vi "Redraw graphs.vi"(6 "Data":sgl[][](array[numeric]), 8 "error in (no error)":errorcluster, 9 "Selected exp":bool=TRUE, 10 "ChangeAll":bool, 11 "Control-Client in":refnum<class "Control-Client.lvclass">) -> (0 "error out":errorcluster, 3 "Control-Client out":refnum<class "Control-Client.lvclass">)   [LabVIEW 2018, in "Control-Client.lvclass"]
uses:
  Control-Client.lvclass
  Control-Client.lvclass/Control-Client.ctl
  Experiments/Experiment.lvclass
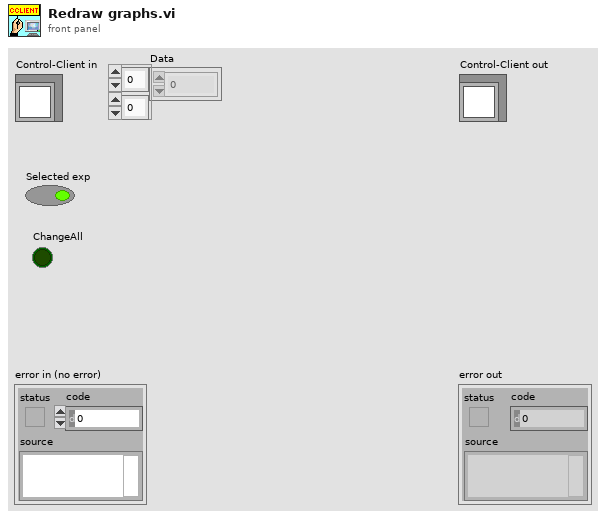
[diagram p1: front panel]
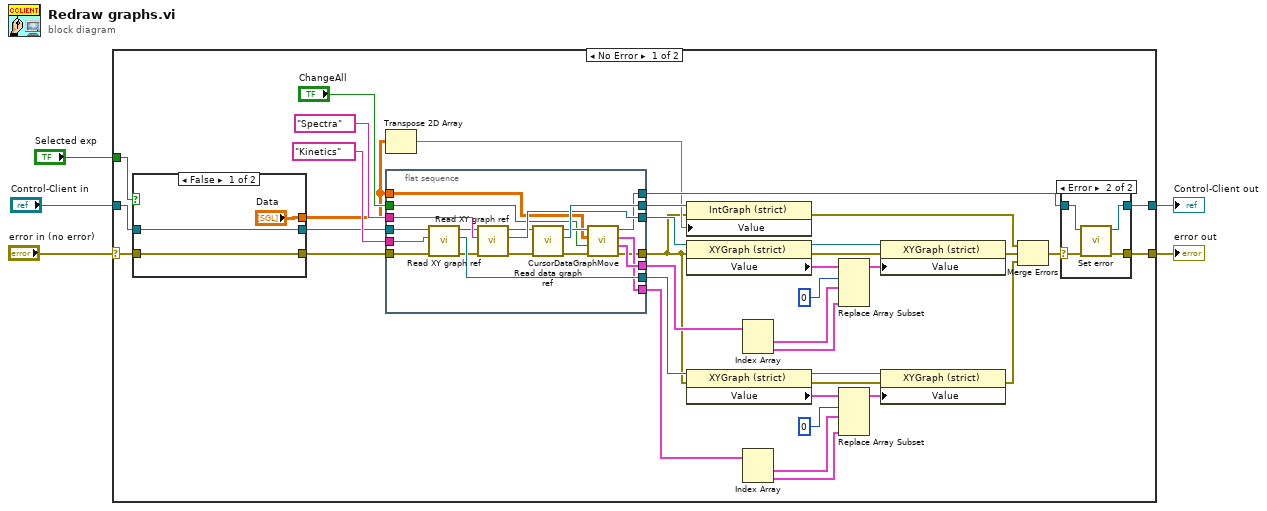
[diagram p0: block diagram]
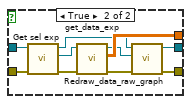
[diagram p2: hidden frame]
diagram:
  n1 = case shown="No Error" "error in (no error)" {
    selector: "error in (no error)" -> [w16 w82]
    tunnel: [w13 w81] -> w3
    tunnel: "Control-Client in" -> [w17 w81]
    tunnel: [w11 w82] -> w2
    tunnel: "Selected exp" -> [w10 _]
    frame No Error {
      n2 = case shown="False" w10 {
        tunnel: w17 -> [w44 w55]
        tunnel: w16 -> [w45 w54]
        tunnel: [w45 w50] -> w6
        tunnel: ["Data" w52] -> w8
        tunnel: [w44 w49] -> w15
        frame False {
        }
        frame True {
          n3 = call "Get sel exp.vi"("error in (no error)"=w54, "Control-Client in"=w55) -> ("error out"=w53:errorcluster, "Sel experiment"=w51:refnum<class "Experiment.lvclass">, "Control-Client out"=w46:refnum<class "Control-Client.lvclass">)  [unwired: 7 in]
          n4 = call "get_data_exp.vi"("error in (no error)"=w53, "Experiment.lvclass in"=w51) -> ("error out"=w47:errorcluster, "Data"=w52:sgl[][], "Experiment.lvclass out"=w48:refnum<class "Experiment.lvclass">)  [unwired: 7 in]
          n5 = call "Redraw_data_raw_graph.vi"("error in (no error)"=w47, "Sel experiment"=w48, "Control-Client in"=w46) -> ("error out"=w50:errorcluster, "Control-Client out"=w49:refnum<class "Control-Client.lvclass">)  [unwired: 7 in]
        }
      }
      n6 = Transpose 2D Array(2D array=w8) -> (transposed array=w9:sgl[][])
      n7 = flat-sequence {
        tunnel: "Kinetics" ("Combo Box") -> [w80]
        tunnel: "Spectra" ("Combo Box") -> [w79]
        tunnel: [w78] -> w40
        tunnel: [w77] -> w39
        tunnel: [w76] -> w38
        tunnel: w15 -> [w62]
        tunnel: w6 -> [w63]
        tunnel: [w75] -> w25
        tunnel: [w74] -> w22
        tunnel: "ChangeAll" -> [w65]
        tunnel: [w70] -> w14
        tunnel: [w66] -> w7
        tunnel: w8 -> [w64]
        frame #0 {
          n8 = call "Read XY graph ref.vi"("error in (no error)"=w63, "Combo Box"=w80, "Control-Client in"=w62) -> ("error out"=w69:errorcluster, "XY graph ref"=w77:refnum<vi>, "Control-Client out"=w73:refnum<class "Control-Client.lvclass">)  [unwired: 6 in]
          n9 = call "Read XY graph ref.vi"("error in (no error)"=w69, "Combo Box"=w79, "Control-Client in"=w73) -> ("error out"=w68:errorcluster, "XY graph ref"=w76:refnum<vi>, "Control-Client out"=w72:refnum<class "Control-Client.lvclass">)  [unwired: 6 in]
          n10 = call "Read data graph ref.vi"("error in (no error)"=w68, "Control-Client in"=w72) -> ("error out"=w67:errorcluster, "Exp data graph ref"=w78:refnum<vi>, "Control-Client out"=w71:refnum<class "Control-Client.lvclass">)  [unwired: 7 in]
          n11 = call "CursorDataGraphMove.vi"("error in (no error)"=w67, "ChangeAll"=w65, "Data"=w64, "Control-Client in"=w71) -> ("error out"=w66:errorcluster, "Spectra"=w75:cluster{"Unités abscisse":dbl[], dbl[]}[], "Kinetics"=w74:cluster{"timedelay":dbl[], dbl[]}[], "Control-Client out"=w70:refnum<class "Control-Client.lvclass">)  [unwired: 2 in, 2 out]
        }
      }
      n12 = property class="IntGraph (strict)"(reference=w40, error in=w7, "Value"=w9) -> (error out=w26:errorcluster)  [unwired: 1 out]
      n13 = property class="XYGraph (strict)"(reference=w38, error in=w7) -> (reference out=w37:refnum<vi>, error out=w36:errorcluster, "Value"=w33:cluster{"Y":dbl[], "Y":dbl[]}[])
      n14 = property class="XYGraph (strict)"(reference=w39, error in=w7) -> (reference out=w35:refnum<vi>, error out=w34:errorcluster, "Value"=w31:cluster{"Y":dbl[], "Y":dbl[]}[])
      n15 = Index Array(array=w25) -> (element #1=w24:cluster{"Unités abscisse":dbl[], dbl[]}, element #2=w23:cluster{"Unités abscisse":dbl[], dbl[]})  [unwired: 2 in]
      n16 = Index Array(array=w22) -> (element #1=w21:cluster{"timedelay":dbl[], dbl[]}, element #2=w20:cluster{"timedelay":dbl[], dbl[]})  [unwired: 2 in]
      n17 = Replace Array Subset(array=w33, new element #1=w24, index #1=0 ("index"), new element #2=w23) -> (w32:cluster{"Y":dbl[], "Y":dbl[]}[])  [unwired: 1 in]
      n18 = Replace Array Subset(array=w31, new element #1=w21, index #1=0 ("index"), new element #2=w20) -> (w30:cluster{"Y":dbl[], "Y":dbl[]}[])  [unwired: 1 in]
      n19 = property class="XYGraph (strict)"(reference=w37, error in=w36, "Value"=w32) -> (error out=w28:errorcluster)  [unwired: 1 out]
      n20 = property class="XYGraph (strict)"(reference=w35, error in=w34, "Value"=w30) -> (error out=w27:errorcluster)  [unwired: 1 out]
      n21 = Merge Errors(w26, w28, w27) -> (w12:errorcluster)
      n22 = case shown="Error" w12 {
        selector: w12 -> [w57 w58]
        tunnel: w14 -> [w56 w61]
        tunnel: [w57 w60] -> w11
        tunnel: [w56 w59] -> w13
        frame No Error {
        }
        frame Error {
          n23 = call "Set error.vi"("error in (no error)"=w58, "Control-Client in"=w61) -> ("error out"=w60:errorcluster, "Control-Client out"=w59:refnum<class "Control-Client.lvclass">)  [unwired: 8 in]
        }
      }
    }
    frame Error {
    }
  }
  "error out" <- w2
  "Control-Client out" <- w3
